vi "PwmConversion.vi"(1 "Invert":bool, 2 "1 to -1 in":dbl) -> (0 "PWM out":u8=128)   [LabVIEW 2013]
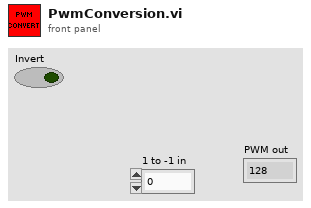
[diagram p1: front panel]
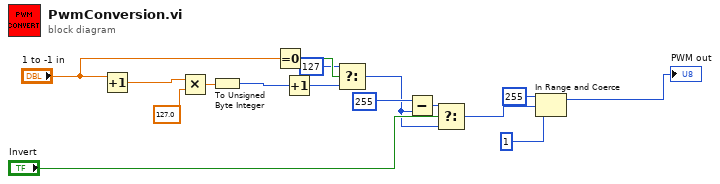
[diagram p0: block diagram]
diagram:
  n1 = Increment(x="1 to -1 in") -> (x+1=w16:dbl)
  n2 = Multiply(x=w16, y=127.0) -> (x*y=w14:dbl)
  n3 = To Unsigned Byte Integer(number=w14) -> (unsigned 8bit integer=w13:u8)
  n4 = Equal To 0?(x="1 to -1 in") -> (x = 0?=w11:bool)
  n5 = Increment(x=w13) -> (x+1=w12:u8)
  n6 = Select(t=u8 127, s=w11, f=w12) -> (s? t:f=w5:u8)
  n7 = Subtract(x=u8 255 ("t"), y=w5) -> (x-y=w7:u8)
  n8 = Select(t=w7, s="Invert", f=w5) -> (s? t:f=w4:u8)
  n9 = In Range and Coerce(upper limit=u8 255, x=w4, lower limit=u8 1) -> (coerced(x)=→"PWM out":u8)  [unwired: 1 out]
